vi "Vi principal_3.vi"() -> ()   [LabVIEW 2017]
uses:
  Control 1.ctl
  Control 2.ctl
  <vilib>/Instr/_visa.llb/VISA Configure Serial Port (Instr).vi
panel:
  out "A":string caption="Actividad"
  in  "NM":T1 caption="Numero de muestra"
  out "T2 2":dbl(slide) caption="Temperatura del liquido" scale=0.0..100.0 scale format="%#_4g"
  in  "c":T1 caption="contador\ncontador"
  in  "SP":i8(slide) caption="Valor deseado" min=0 max=100 scale=0.0..100.0
  out "T1":dbl(slide) caption="Temperatura ambiente" scale=0.0..100.0 scale format="%#_4g"
  out "T2":dbl(slide) caption="Temperatura del liquido" scale=0.0..100.0 scale format="%#.1f"
  out "G":cluster{"SP":i8, "T1":dbl}(graph)={"SP"=18, "T1"=21.125} caption="Grafico de Temperatura (C*)"
  in  "R/w":enum16{"read/write", "read-only", "write-only"}(ring) caption="Accion en Archivo"
  in  "RA":path caption="Ruta de Archivo"
  in  "VISA resource name":T2
  in  "A":bool caption="Arranque"
  in  "P":bool caption="Paro"
  # "Grados C*"
  # "Grados C*"
  # "Grados C*"
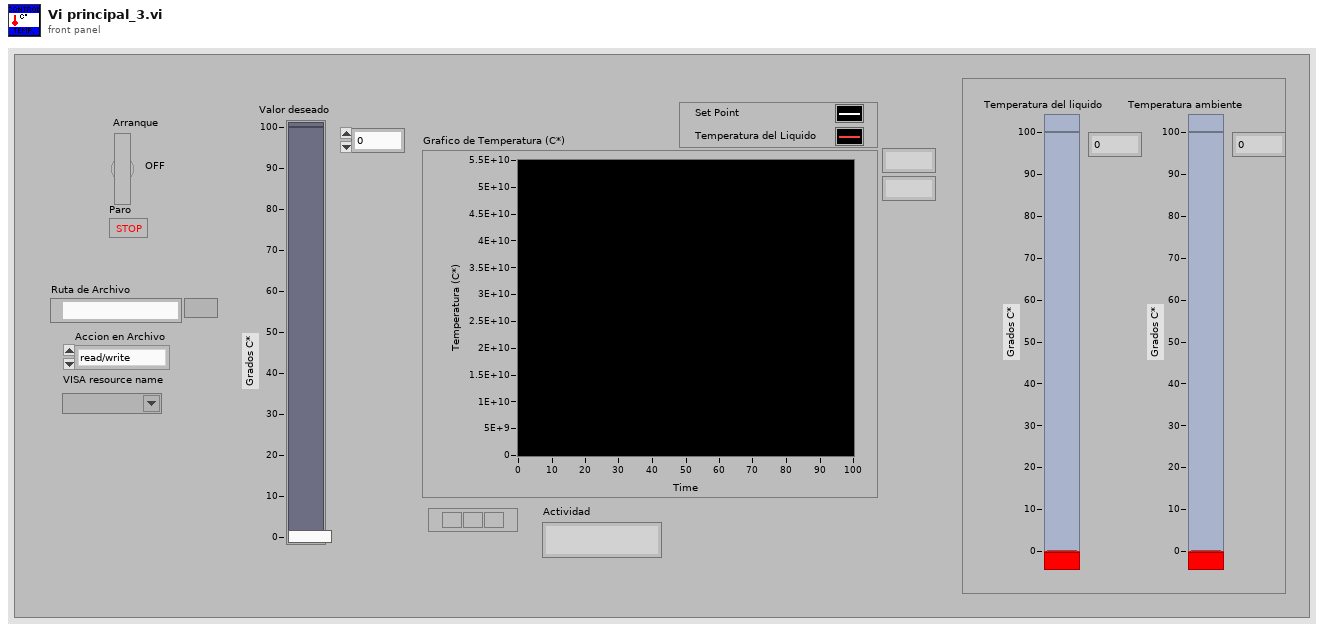
[diagram p1: front panel]
types:
  T1 = typedef "Control 2.ctl" = u8
  T2 = typedef "Control 1.ctl" = refnum<visa-resource-name>
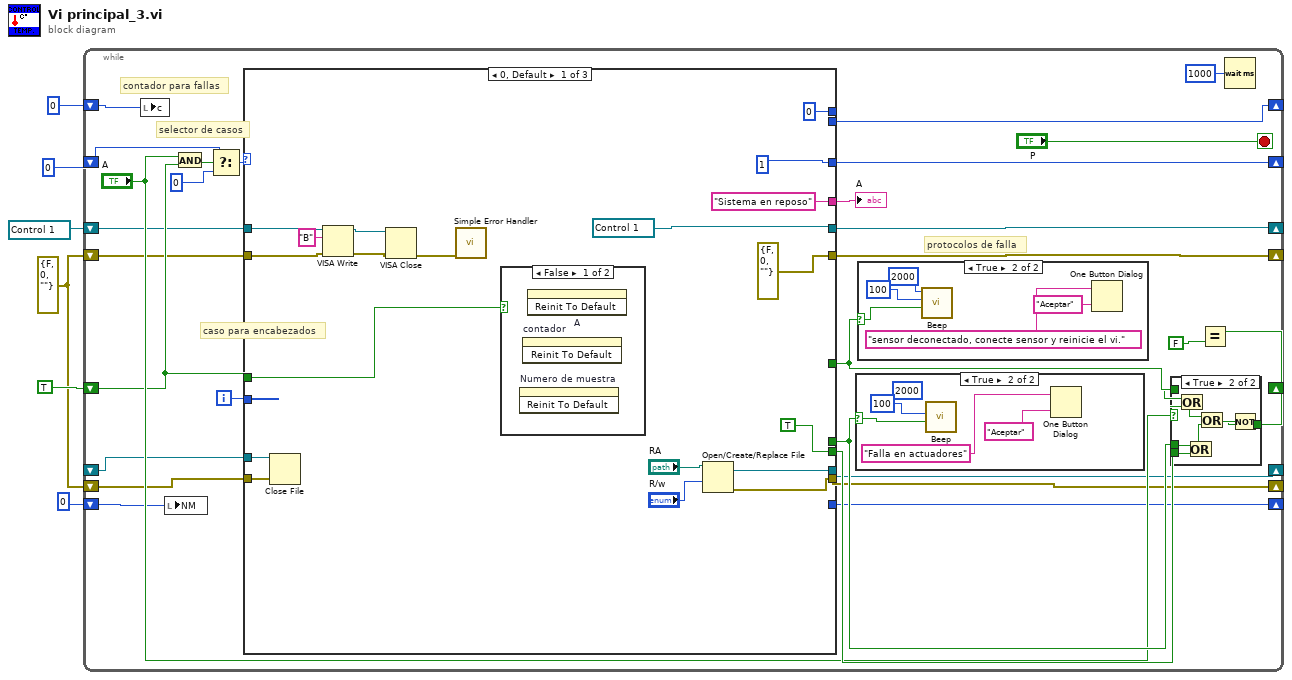
[diagram p0: block diagram]
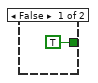
[diagram p2: hidden frame]
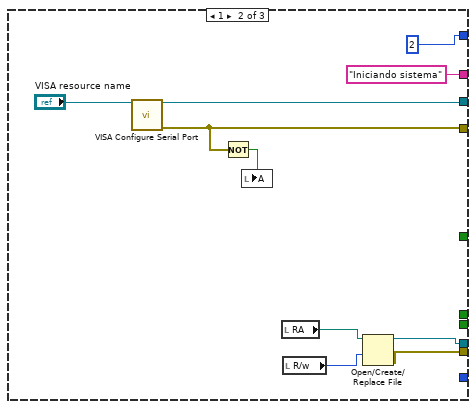
[diagram p6: hidden frame]
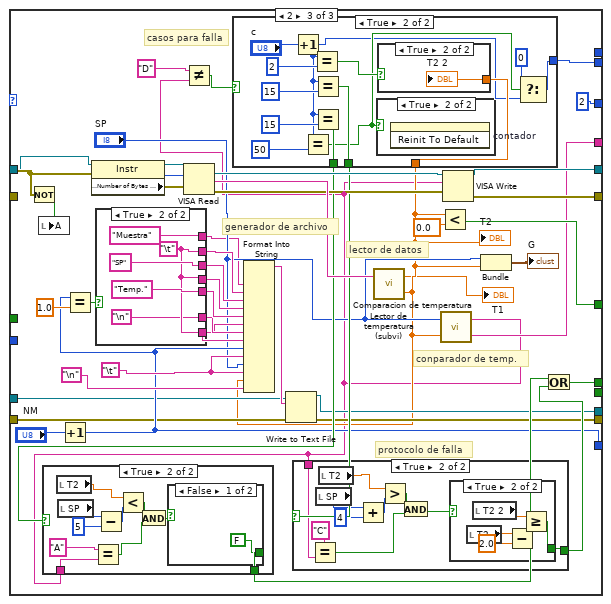
[diagram p7: hidden frame]
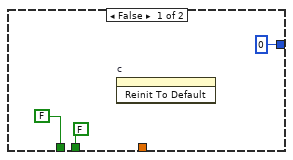
[diagram p8: hidden frame]
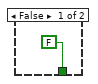
[diagram p11: hidden frame]
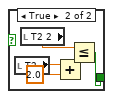
[diagram p12: hidden frame]
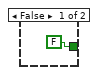
[diagram p13: hidden frame]
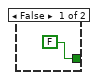
[diagram p14: hidden frame]
diagram:
  w1 = errorcluster {"status"=FALSE, "code"=0, "source"=""} ("error out")
  n1 = while {
    shift-right: [w11] -> _
    shift-left: TRUE -> [w27]
    shift-right: [w25] -> _
    shift-left: 0 -> [w22]
    shift-right: [w10] -> _
    shift-left: w1 -> [w21]
    shift-right: [w9] -> _
    shift-left: T2 "COM3" ("VISA resource name") -> [w13]
    shift-right: [w7] -> _
    shift-left: 0 -> [w20]
    shift-right: [w19] -> _
    shift-left: 0 -> [w18]
    shift-right: [w15] -> _
    shift-left: _ -> [w16]
    shift-right: [w14] -> _
    shift-left: w1 -> [w17]
    i -> [w29]
    stop <- "P" stop-if-true
    # "caso para encabezados"
    # "contador para fallas"
    # "protocolos de falla"
    # "selector de casos"
    n2 = local write "c"(w20) -> ()
    n3 = local write "NM"(w18) -> ()
    n4 = And(x="A", y=w27) -> (x .and. y?=w24:bool)
    n5 = Select(t=w22, s=w24, f=0) -> (s? t:f=w23:i32)
    n6 = case shown="0, Default" w23 {
      tunnel: [_ _ w100] -> w33
      tunnel: [_ _ w124] -> w32
      tunnel: [TRUE _ _] -> w31
      tunnel: w29 -> [_ _ _]
      tunnel: w27 -> [w69 _ _]
      tunnel: [1 2 2] -> w25
      tunnel: [T2 "COM3" ("VISA resource name") w78 w106] -> w9
      tunnel: [errorcluster {"status"=FALSE, "code"=0, "source"=""} ("error out") w76 w105] -> w10
      tunnel: w21 -> [w62 _ w104]
      tunnel: [T1 0 _ _] -> _
      tunnel: [_ _ w95] -> w19
      tunnel: w16 -> [w58 _ w94]
      tunnel: w17 -> [w57 _ w93]
      tunnel: [w55 w74 w92] -> w15
      tunnel: [w56 w73 w91] -> w14
      tunnel: w13 -> [w63 _ w90]
      tunnel: ["Sistema en reposo" ("A") "Iniciando sistema" ("A") w88] -> w8
      tunnel: [_ _ w85] -> w7
      frame 0, Default {
        n7 = Close File(refnum=w58, error in=w57) -> ()  [unwired: 2 out]
        n8 = VISA Write(VISA resource name=w63, write buffer="B", error in (no error)=w62) -> (VISA resource name out=w64:T2, error out=w65:errorcluster)  [unwired: 1 out]
        n9 = VISA Close(VISA resource name=w64, error in (no error)=w65) -> (error out=w66:errorcluster)
        n10 = call <vilib>:"Simple Error Handler.vi"("error in (no error)"=w66) -> ()  [unwired: 4 in, 5 out]
        n11 = case shown="False" w69 {
          frame False {
            n12 = invoke on="Numero de muestra" class="DigNum (strict)" method="Reinit To Default"() -> ()  [unwired: 3 in, 3 out]
            n13 = invoke on="contador" class="DigNum (strict)" method="Reinit To Default"() -> ()  [unwired: 3 in, 3 out]
            n14 = invoke on="A" class="Bool (strict)" method="Reinit To Default"() -> ()  [unwired: 3 in, 3 out]
          }
          frame True {
          }
        }
        n15 = Open/Create/Replace File(file path (use dialog)="RA", access (0:read/write)="R/w") -> (refnum out=w55:refnum<file>, error out=w56:errorcluster)  [unwired: 4 in, 1 out]
      }
      frame 1 {
        n16 = call-poly "VISA Configure Serial Port"("VISA resource name"="VISA resource name") -> ("VISA resource name out"=w78:refnum<visa-resource-name>, "error out"=w76:errorcluster)  [unwired: 13 in]
        n17 = Not(x=w76) -> (.not. x?=w77:bool)
        n18 = local write "A"(w77) -> ()
        n19 = local read "RA"() -> (w71:path)
        n20 = local read "R/w"() -> (w72:enum16{"read/write", "read-only", "write-only"})
        n21 = Open/Create/Replace File(file path (use dialog)=w71, access (0:read/write)=w72) -> (refnum out=w74:refnum<file>, error out=w73:errorcluster)  [unwired: 4 in, 1 out]
      }
      frame 2 {
        w120 = "\t"
        # "casos para falla"
        # "protocolo de falla"
        # "lector de datos"
        # "conparador de temp."
        # "generador de archivo"
        n22 = Not(x=w104) -> (.not. x?=w103:bool)
        n23 = local write "A"(w103) -> ()
        n24 = Increment(x="NM") -> (x+1=w95:T1)
        n25 = Equal?(x=w95, y=1.0) -> (x = y?=w122:bool)
        n26 = property class="Instr"(reference=w90, error in=w104) -> (reference out=w113:T2, error out=w111:errorcluster, "Serial Settings:Number of Bytes at Serial Port"=w112:u32)
        n27 = case shown="True" w122 {
          tunnel: [_ "Muestra"] -> w81
          tunnel: [_ "SP"] -> w118
          tunnel: [_ "Temp."] -> w116
          tunnel: [_ w179] -> w119
          tunnel: [_ w179] -> w117
          tunnel: [_ "\n"] -> w115
          tunnel: [_ w179] -> w114
          frame False {
          }
          frame True {
            w179 = "\t"
          }
        }
        n28 = VISA Read(VISA resource name=w113, byte count=w112, error in (no error)=w111) -> (VISA resource name out=w108:T2, read buffer=w110:string, error out=w107:errorcluster)  [unwired: 1 out]
        n29 = call "Lector de temperatura (subvi).vi"("read buffer"=w110) -> ("T1"=w87:dbl, "T2"=→"T1":dbl)  [unwired: 1 in]
        "T2" <- w87
        n30 = Format Into String(w81, w119, w118, w117, w116, w114, w115, w114, w95, w120, "SP", w120, w87, "\n") -> (resulting string=w123:string)  [unwired: 3 in, 1 out]
        n31 = Write to Text File(file (use dialog)=w94, text=w123, error in=w93) -> (refnum out=w92:refnum<file>, error out=w91:errorcluster)  [unwired: 1 in, 1 out]
        n32 = Less?(x=w87, y=0.0 ("x")) -> (x < y?=w124:bool)
        n33 = call "Comparacion de temperatura.vi"("T2"=w87, "SP"="SP") -> ("A"=w88:string, "C"=w82:string)
        n34 = Not Equal?(x="D", y=w82) -> (x != y?=w83:bool)
        n35 = case shown="True" w83 {
          tunnel: [FALSE w139] -> w101
          tunnel: [FALSE w137] -> w97
          tunnel: w87 -> [_ w134]
          tunnel: [T1 0 w131] -> w85
          frame False {
            n36 = invoke on="c" class="DigNum (strict)" method="Reinit To Default"() -> ()  [unwired: 3 in, 3 out]
          }
          frame True {
            n37 = Increment(x="c") -> (x+1=w132:T1)
            n38 = Equal?(x=w132, y=u8 50) -> (x = y?=w135:bool)
            n39 = Equal?(x=w132, y=u8 2) -> (x = y?=w142:bool)
            n40 = Equal?(x=w132, y=u8 15) -> (x = y?=w139:bool)
            n41 = Equal?(x=w132, y=u8 15) -> (x = y?=w137:bool)
            n42 = case shown="True" w135 {
              frame False {
              }
              frame True {
                n43 = invoke on="contador" class="DigNum (strict)" method="Reinit To Default"() -> ()  [unwired: 3 in, 3 out]
              }
            }
            n44 = case shown="True" w142 {
              tunnel: w134 -> [_ w143]
              frame False {
              }
              frame True {
                "T2 2" <- w143
              }
            }
            n45 = Select(t=u8 0, s=w135, f=w132) -> (s? t:f=w131:T1)
          }
        }
        n46 = case shown="True" w97 {
          tunnel: w82 -> [_ w154]
          tunnel: [FALSE w152] -> w98
          frame False {
          }
          frame True {
            n47 = local read "T2"() -> (w148:dbl)
            n48 = local read "SP"() -> (w146:i8)
            n49 = Equal?(x="A", y=w154) -> (x = y?=w149:bool)
            n50 = Subtract(x=w146, y=u8 5) -> (x-y=w147:u8)
            n51 = Less?(x=w148, y=w147) -> (x < y?=w150:bool)
            n52 = And(x=w150, y=w149) -> (x .and. y?=w151:bool)
            n53 = case shown="False" w151 {
              tunnel: [FALSE w159] -> w152
              frame False {
              }
              frame True {
                n54 = local read "T2"() -> (w157:dbl)
                n55 = local read "T2 2"() -> (w160:dbl)
                n56 = Add(x=w157, y=2.0) -> (x+y=w158:dbl)
                n57 = Less Or Equal?(x=w160, y=w158) -> (x <= y?=w159:bool)
              }
            }
          }
        }
        n58 = case shown="True" w101 {
          tunnel: w82 -> [_ w171]
          tunnel: [FALSE w169] -> w99
          frame False {
          }
          frame True {
            n59 = Equal?(x="C", y=w171) -> (x = y?=w163:bool)
            n60 = local read "SP"() -> (w167:i8)
            n61 = local read "T2"() -> (w162:dbl)
            n62 = Add(x=w167, y=u8 4) -> (x+y=w166:u8)
            n63 = Greater?(x=w162, y=w166) -> (0:w165:bool)
            n64 = And(x=w165, y=w163) -> (x .and. y?=w164:bool)
            n65 = case shown="True" w164 {
              tunnel: [FALSE w176] -> w169
              frame False {
              }
              frame True {
                n66 = local read "T2"() -> (w174:dbl)
                n67 = local read "T2 2"() -> (w177:dbl)
                n68 = Subtract(x=w174, y=2.0) -> (x-y=w175:dbl)
                n69 = Greater Or Equal?(x=w177, y=w175) -> (x >= y?=w176:bool)
              }
            }
          }
        }
        n70 = VISA Write(VISA resource name=w108, write buffer=w82, error in (no error)=w107) -> (VISA resource name out=w106:T2, error out=w105:errorcluster)  [unwired: 1 out]
        n71 = Bundle("SP"="SP", "T1"=w87) -> (→"G":cluster{"SP":i8, "T1":dbl})  [unwired: 1 in]
        n72 = Or(x=w98, y=w99) -> (x .or. y?=w100:bool)
      }
    }
    "A" <- w8
    n73 = case shown="True" w33 {
      selector: w33 -> [_ w49]
      frame False {
      }
      frame True {
        (unwired) u32 2000 ("frequency (Hz)")
        n74 = call <vilib>:"Beep.vi"("use system alert? (T)"=w49, "duration (msec)"=u32 100) -> ()  [unwired: 10 in]
        n75 = One Button Dialog(message="Falla en actuadores", button name ("OK")="Aceptar") -> ()  [unwired: 1 out]
      }
    }
    n76 = case shown="True" w32 {
      selector: w32 -> [_ w46]
      frame False {
      }
      frame True {
        n77 = call <vilib>:"Beep.vi"("use system alert? (T)"=w46, "duration (msec)"=u32 100, "frequency (Hz)"=u32 2000) -> ()  [unwired: 9 in]
        n78 = One Button Dialog(message="sensor deconectado, conecte sensor y reinicie el vi.", button name ("OK")="Aceptar") -> ()  [unwired: 1 out]
      }
    }
    n79 = case shown="True" "A" {
      tunnel: [TRUE w41] -> w11
      tunnel: w33 -> [_ w38]
      tunnel: w32 -> [_ w37]
      tunnel: w31 -> [_ w36]
      frame False {
      }
      frame True {
        n80 = Or(x=w37, y=w36) -> (x .or. y?=w40:bool)
        n81 = Or(x=w38, y=w36) -> (x .or. y?=w39:bool)
        n82 = Or(x=w40, y=w39) -> (x .or. y?=w42:bool)
        n83 = Not(x=w42) -> (.not. x?=w41:bool)
      }
    }
    n84 = Equal?(x=w11, y=FALSE) -> ()  [unwired: 1 out]
    n85 = Wait (ms)(milliseconds to wait=u32 1000) -> ()  [unwired: 1 out]
  }
